vi "华氏转摄氏.vi"(10 "Numeric 2":dbl) -> (2 "Numeric":dbl)   [LabVIEW 2020]
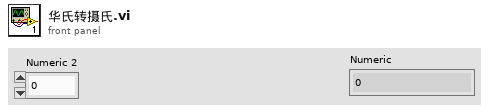
[diagram p1: front panel]
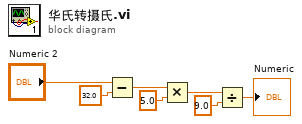
[diagram p0: block diagram]
diagram:
  n1 = Subtract(x="Numeric 2", y=32.0) -> (x-y=w6:dbl)
  n2 = Multiply(x=w6, y=5.0) -> (x*y=w4:dbl)
  n3 = Divide(x=w4, y=9.0) -> (x/y=→"Numeric":dbl)
